vi "pullNodeFromOpen.vi"(8 "error in (no error)":errorcluster, 11 "Tree in":refnum<class "Tree.lvclass">) -> (0 "error out":errorcluster, 1 "empty":bool, 2 "RemovedNode":refnum<data-value>, 3 "Tree out":refnum<class "Tree.lvclass">)   [LabVIEW 2010, in "Tree.lvclass"]
doc: "Pulls the first node from the sorted list open. The first node represents the node we think is most likely to be the goal node."
uses:
  Tree.lvclass
  TreeNode/TreeNode.lvclass
  Tree.lvclass/Tree.ctl
  LinkedList/position.ctl
  LinkedList/LinkedList.lvclass
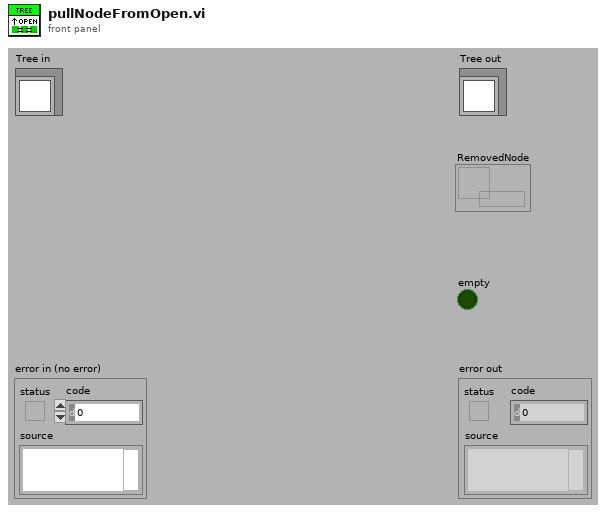
[diagram p1: front panel]
types:
  T1 = typedef "LinkedList.lvclass/position.ctl" = enum16{"Front", "Back", "Search"}
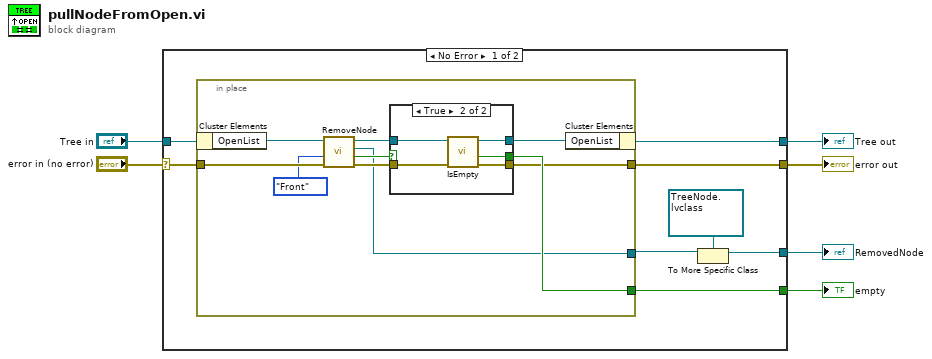
[diagram p0: block diagram]
diagram:
  n1 = case shown="No Error" "error in (no error)" {
    selector: "error in (no error)" -> [w13 w33]
    tunnel: [w10 w33] -> w5
    tunnel: [w11 w32] -> w3
    tunnel: "Tree in" -> [w14 w32]
    tunnel: [w12 _] -> w2
    tunnel: [w7 _] -> w1
    frame No Error {
      n2 = in-place {
        in-place-border: w13 -> [w23]
        in-place-border: [w18] -> w12
        in-place-border: [w17] -> w9
        in-place-border: [w15] -> w10
        n3 = in-place-cluster #1(w14) -> ("OpenList"=w24:refnum<class "BasicSortedList.lvclass">)
        n4 = call "RemoveNode.vi"("error in (no error)"=w23, "position"=position."Front", "LinkedList in"=w24) -> ("error out"=w19:errorcluster, "ignored"=w20:bool, "RemovedNode"=w17:refnum<data-value>, "LinkedList out"=w21:refnum<class "BasicSortedList.lvclass">)  [unwired: 5 in]
        n5 = case shown="True" w20 {
          tunnel: w21 -> [w26 w31]
          tunnel: w19 -> [w25 w30]
          tunnel: [_ w29] -> w18
          tunnel: [w26 w28] -> w16
          tunnel: [w25 w27] -> w15
          frame False {
          }
          frame True {
            n6 = call "IsEmpty.vi"("error in (no error)"=w30, "LinkedList in"=w31) -> ("error out"=w27:errorcluster, "empty"=w29:bool, "LinkedList out"=w28:refnum<class "BasicSortedList.lvclass">)  [unwired: 7 in]
          }
        }
        n7 = in-place-cluster #1("OpenList"=w16) -> (w11:refnum<class "Tree.lvclass">)
      }
      n8 = To More Specific Class(target class=refnum<data-value> refnum ("data value reference"), reference=w9) -> (specific class reference=w7:refnum<data-value>)  [unwired: 1 in, 1 out]
    }
    frame Error {
    }
  }
  "error out" <- w5
  "Tree out" <- w3
  "empty" <- w2
  "RemovedNode" <- w1
